vi "PC.vi"() -> ()   [LabVIEW 2021]
uses:
  <resource>/objmgr/ni.dex.rc
panel:
  in  "Message to send":i32[](array[numeric])
  in  "Send":bool
  in  "stop":bool
  out "RT Connected?":bool
  in  "myRIO IP Address":string
  out "RT reader URL":string
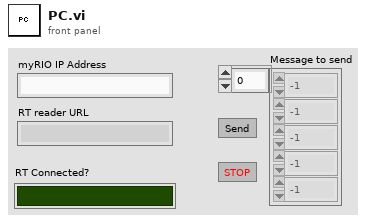
[diagram p1: front panel]
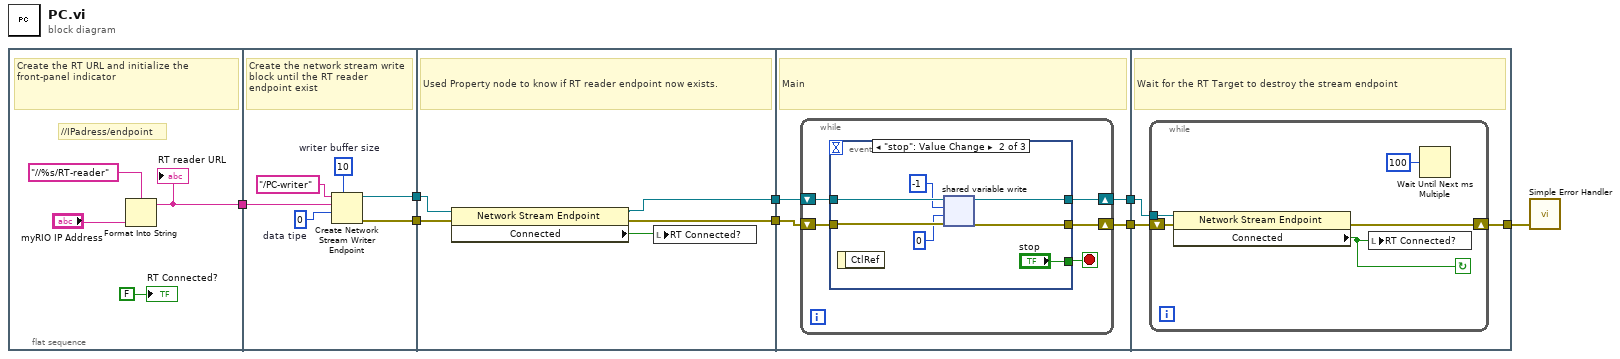
[diagram p0: block diagram]
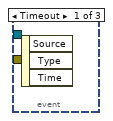
[diagram p2: hidden frame]
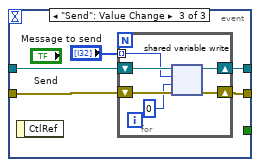
[diagram p3: hidden frame]
diagram:
  n1 = flat-sequence {
    tunnel: [w12] -> w8
    tunnel: w8 -> [w18]
    tunnel: [w14] -> w7
    tunnel: [w13] -> w6
    tunnel: w7 -> [w21]
    tunnel: w6 -> [w23]
    tunnel: [w22] -> w5
    tunnel: [w19] -> w4
    tunnel: w5 -> [w26]
    tunnel: w4 -> [w27]
    tunnel: [w25] -> w3
    tunnel: [w24] -> w2
    tunnel: [w52] -> w1
    tunnel: w3 -> [w51]
    tunnel: w2 -> [w53]
    frame #0 {
      # "//IPadress/endpoint"
      # "Create the RT URL and initialize the front-panel indicator"
      n2 = Format Into String(format string="//%s/RT-reader", "myRIO IP Address") -> (resulting string=w12:string)  [unwired: 2 in, 1 out]
      "RT reader URL" <- w12
      "RT Connected?" <- FALSE ("RT Connected?")
    }
    frame #1 {
      w15 = 0  # data tipe
      w16 = 10  # writer buffer size
      # "Create the network stream write block until the RT reader endpoint exist"
      n3 = Create Network Stream Writer Endpoint(7:w16, 9:w15, 10:w18, 11:"/PC-writer" ("writer name")) -> (0:w13:errorcluster, 3:w14:refnum<k21>)  [unwired: 3 in]
    }
    frame #2 {
      # "Used Property node to know if RT reader endpoint now exists."
      n4 = property class="Network Stream Endpoint"(reference=w21, error in=w23) -> (reference out=w19:refnum<k21>, error out=w22:errorcluster, "Connected"=w20:bool)
      n5 = local write "RT Connected?"(w20) -> ()
    }
    frame #3 {
      # "Main"
      n6 = while {
        shift-right: [w29] -> w25
        shift-left: w27 -> [w32]
        shift-right: [w28] -> w24
        shift-left: w26 -> [w31]
        stop <- w30 stop-if-true
        n7 = event shown="[1] \"stop\": Value Change" {
          selector: _ -> [_ _ _]
          dyn-events: _ -> [_ _ _]
          timeout: _ -> [_ _ _]
          tunnel: w32 -> [_ w38 w44]
          tunnel: w31 -> [_ w35 w41]
          tunnel: [_ "stop" _] -> w30
          tunnel: [_ w37 w43] -> w29
          tunnel: [_ w36 w42] -> w28
          event Timeout {
            n8 = event-data() -> ()  [unwired: 1 in, 3 out]
          }
          event "stop": Value Change {
            n9 = event-data() -> ()  [unwired: 1 in, 1 out]
            n10 = shared-variable-write(w38, w35, -1 ("data in"), 0 ("timeout ms (-1)")) -> (w37:refnum<k21>, w36:errorcluster)  [unwired: 1 out]
          }
          event "Send": Value Change {
            n11 = event-data() -> ()  [unwired: 1 in, 1 out]
            n12 = for {
              tunnel: "Message to send" -> [w45] mode=indexing
              shift-right: [w49] -> w43
              shift-left: w44 -> [w50]
              shift-right: [w48] -> w42
              shift-left: w41 -> [w47]
              n13 = shared-variable-write(w50, w47, w45, 0 ("timeout ms (-1)")) -> (w49:refnum<k21>, w48:errorcluster)  [unwired: 1 out]
            }
          }
        }
      }
    }
    frame #4 {
      # "Wait for the RT Target to destroy the stream endpoint"
      n14 = while {
        tunnel: w51 -> [w56]
        shift-right: [w57] -> w52
        shift-left: w53 -> [w58]
        stop <- w55 continue-if-true
        n15 = property class="Network Stream Endpoint"(reference=w56, error in=w58) -> (error out=w57:errorcluster, "Connected"=w55:bool)  [unwired: 1 out]
        n16 = local write "RT Connected?"(w55) -> ()
        n17 = Wait Until Next ms Multiple(millisecond multiple=u32 100) -> ()  [unwired: 1 out]
      }
    }
  }
  n18 = call <vilib>:"Simple Error Handler.vi"("error in (no error)"=w1) -> ()  [unwired: 4 in, 5 out]
